vi "accelerometer.vi"() -> ()   [LabVIEW 2020]
uses:
  <vilib>/DAQmx/read.llb/DAQmx Read (Analog 1D Wfm NChan NSamp).vi
  <vilib>/DAQmx/create/channels.llb/DAQmx Create Channel (AI-Acceleration-Accelerometer).vi
  <vilib>/DAQmx/configure/timing.llb/DAQmx Timing (Sample Clock).vi
  <vilib>/DAQmx/miscellaneous.llb/DAQmx Fill In Error Info.vi
  <resource>/objmgr/daqmx.rc
panel:
  out "data":dynamicdata(graph)
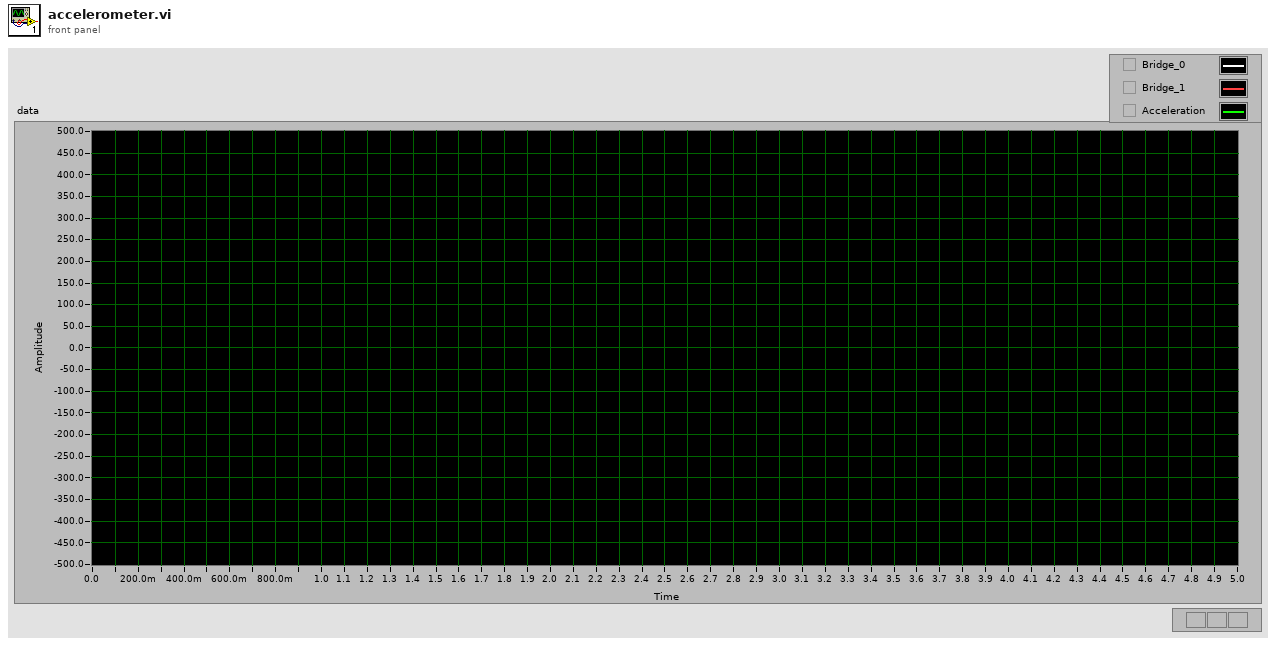
[diagram p1: front panel]
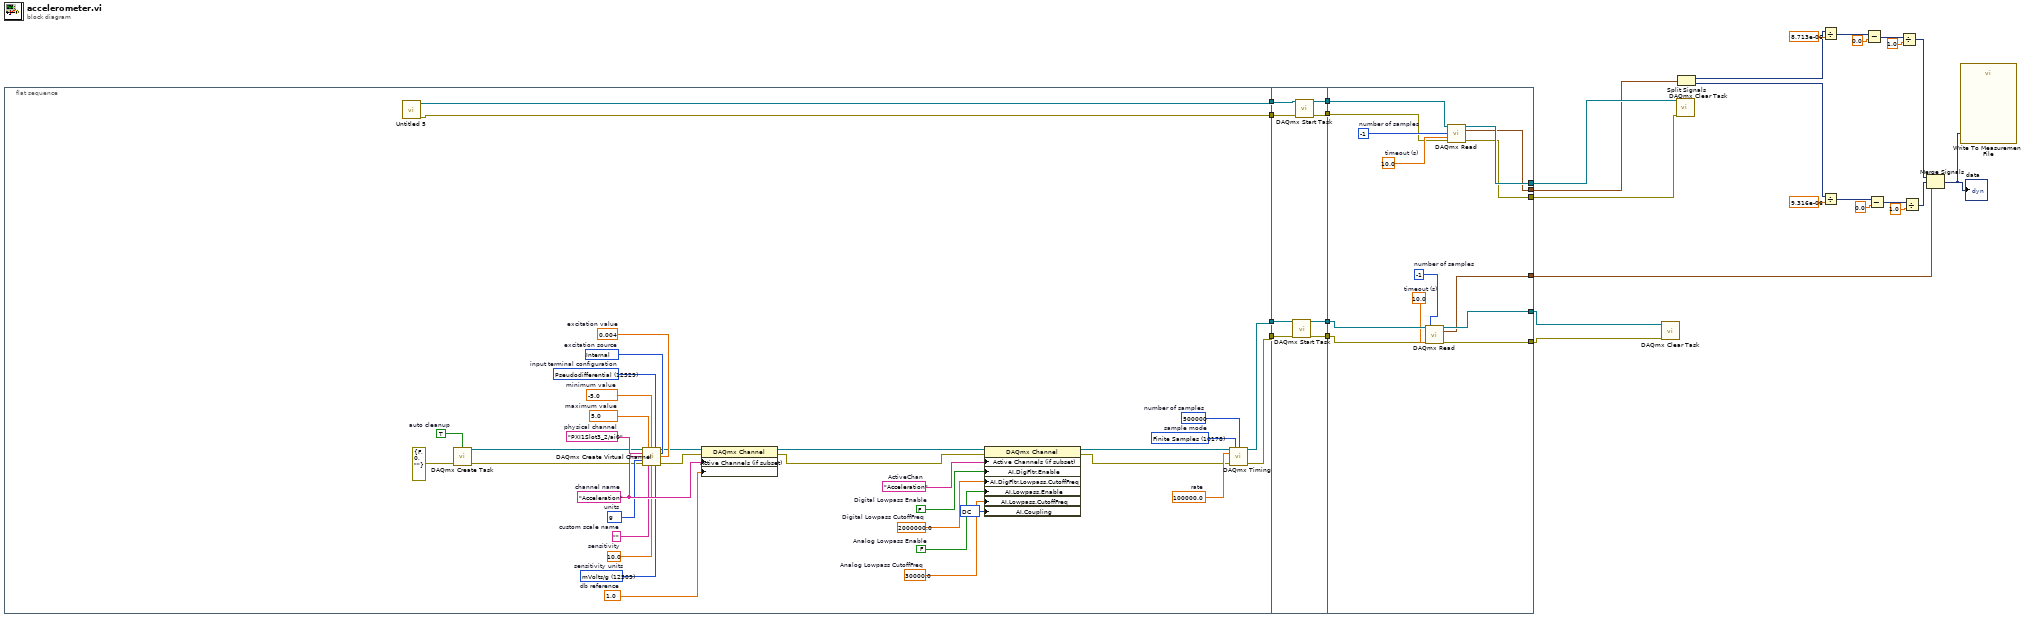
[diagram p0: block diagram]
diagram:
  n1 = flat-sequence {
    tunnel: [w61] -> w21
    tunnel: [w62] -> w20
    tunnel: [w63] -> w19
    tunnel: [w64] -> w18
    tunnel: w21 -> [w72]
    tunnel: w20 -> [w71]
    tunnel: w19 -> [w66]
    tunnel: w18 -> [w65]
    tunnel: [w70] -> w17
    tunnel: [w69] -> w16
    tunnel: [w68] -> w15
    tunnel: [w67] -> w14
    tunnel: w17 -> [w79]
    tunnel: w16 -> [w76]
    tunnel: w15 -> [w86]
    tunnel: w14 -> [w83]
    tunnel: [w82] -> w13
    tunnel: [w81] -> w12
    tunnel: [w80] -> w11
    tunnel: [w75] -> w10
    tunnel: [w74] -> w9
    tunnel: [w73] -> w8
    frame #0 {
      w30 = 10050 items=["AC"=10045, "DC"=10050, "GND"=10066] ("AI.Coupling")
      w59 = 10178 items=["Finite Samples"=10178, "Continuous Samples"=10123, "Hardware Timed Single Point"=12522]  # sample mode
      w58 = 500000  # number of samples
      w57 = 100000.0  # rate
      w55 = 30000.0  # Analog Lowpass CutoffFreq
      w54 = FALSE  # Analog Lowpass Enable
      w53 = 2000000.0  # Digital Lowpass CutoffFreq
      w51 = FALSE  # Digital Lowpass Enable
      w49 = "Acceleration"  # ActiveChan
      w47 = 1.0  # db reference
      w44 = 10186 items=["g"=10186, "m/s^2"=12470, "From Custom Scale"=10065]  # units
      w43 = 12529 items=["default"=-1, "RSE"=10083, "NRSE"=10078, "Differential"=10106, "Pseudodifferential"=12529]  # input terminal configuration
      w42 = 10200 items=["Internal"=10200, "External"=10167, "None"=10230]  # excitation source
      w41 = 0.004  # excitation value
      w40 = 12509 items=["mVolts/g"=12509, "Volts/g"=12510]  # sensitivity units
      w39 = 10.0  # sensitivity
      w48 = "Acceleration"  # channel name
      w37 = ""  # custom scale name
      w36 = -5.0  # minimum value
      w35 = 5.0  # maximum value
      w34 = "PXI1Slot3_2/ai0"  # physical channel
      w32 = TRUE  # auto cleanup
      n2 = call "Untitled 5.vi"() -> ("error out"=w64:errorcluster, "task out"=w63:refnum<k21>)  [unwired: 10 in]
      n3 = call <vilib>:"DAQmx Create Task.vi"("auto cleanup"=w32, "error in"=errorcluster {"status"=FALSE, "code"=0, "source"=""}) -> ("task out"=w33:refnum<k21>, "error out"=w31:errorcluster)  [unwired: 12 in]
      n4 = call-poly <vilib>:"DAQmx Create Virtual Channel.vi"("task in"=w33, "maximum value"=w35, "minimum value"=w36, "input terminal configuration"=w43, "physical channels"=w34, "current excitation source"=w42, "name to assign"=w48, "current excitation value"=w41, "units"=w44, "error in"=w31, "custom scale name"=w37, "sensitivity"=w39, "sensitivity units"=w40) -> ("task out"=w38:refnum<k21>, "error out"=w45:errorcluster)  [unwired: 1 in]
      n5 = property class="DAQmx Channel"(reference=w38, error in=w45, "Active Channels (if subset)"=w48, "Analog Input:Acceleration:dB Reference"=w47) -> (reference out=w52:refnum<k21>, error out=w46:errorcluster)
      n6 = property class="DAQmx Channel"(reference=w52, error in=w46, "Active Channels (if subset)"=w49, "AI.DigFltr.Enable"=w51, "AI.DigFltr.Lowpass.CutoffFreq"=w53, "AI.Lowpass.Enable"=w54, "AI.Lowpass.CutoffFreq"=w55, "AI.Coupling"=w30) -> (reference out=w56:refnum<k21>, error out=w50:errorcluster)
      n7 = call-poly <vilib>:"DAQmx Timing.vi"("task/channels in"=w56, "sample mode"=w59, "samples per channel"=w58, "rate"=w57, "error in"=w50) -> ("task out"=w61:refnum<k21>, "error out"=w62:errorcluster)  [unwired: 9 in]
    }
    frame #1 {
      n8 = call <vilib>:"DAQmx Start Task.vi"("task/channels in"=w72, "error in"=w71) -> ("task out"=w70:refnum<k21>, "error out"=w69:errorcluster)  [unwired: 12 in]
      n9 = call <vilib>:"DAQmx Start Task.vi"("task/channels in"=w66, "error in"=w65) -> ("task out"=w68:refnum<k21>, "error out"=w67:errorcluster)  [unwired: 12 in]
    }
    frame #2 {
      w77 = 10.0  # timeout (s)
      w78 = -1  # number of samples
      w84 = 10.0  # timeout (s)
      w85 = -1  # number of samples
      n10 = call-poly <vilib>:"DAQmx Read.vi"("task/channels in"=w79, "number of samples per channel"=w78, "timeout"=w77, "error in"=w76) -> ("task out"=w75:refnum<k21>, "data"=w74:waveform(dbl)[], "error out"=w73:errorcluster)  [unwired: 9 in]
      n11 = call-poly <vilib>:"DAQmx Read.vi"("task/channels in"=w86, "number of samples per channel"=w85, "timeout"=w84, "error in"=w83) -> ("task out"=w82:refnum<k21>, "data"=w81:waveform(dbl)[], "error out"=w80:errorcluster)  [unwired: 9 in]
    }
  }
  n12 = call <vilib>:"DAQmx Clear Task.vi"("task in"=w10, "error in"=w8) -> ()  [unwired: 13 in, 1 out]
  n13 = call <vilib>:"DAQmx Clear Task.vi"("task in"=w13, "error in"=w11) -> ()  [unwired: 13 in, 1 out]
  n14 = Split Signals(w12) -> (w23:dynamicdata, w22:dynamicdata)  [unwired: 2 in]
  n15 = Divide(x=w23, y=8.713e-06) -> (x/y=w25:dynamicdata)
  n16 = Divide(x=w22, y=9.316e-06) -> (x/y=w24:dynamicdata)
  n17 = Subtract(x=w25, y=0.0) -> (x-y=w5:dynamicdata)
  n18 = Subtract(x=w24, y=0.0) -> (x-y=w7:dynamicdata)
  n19 = Divide(x=w5, y=1.0) -> (x/y=w3:dynamicdata)
  n20 = Divide(x=w7, y=1.0) -> (x/y=w2:dynamicdata)
  n21 = Merge Signals(w3, w2, w9) -> (w1:dynamicdata)
  "data" <- w1
  n22 = call "Write To Measurement File"("Signals"=w1) -> ()  [unwired: 16 in, 3 out]
